vi "RT-Main.vi"   [LabVIEW 2019]
uses:
  <vilib>/nisyscfg/Close (System).vi
  <vilib>/nisyscfg/nisyscfg.lvlib
  <vilib>/NI_Real-Time Target Support.lvlib
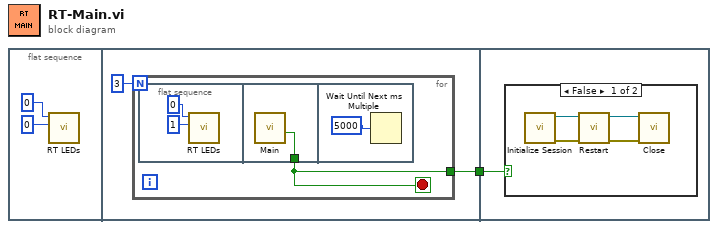
[diagram p0: block diagram]
diagram:
  n1 = flat-sequence {
    tunnel: [w4] -> w1
    tunnel: w1 -> [w11]
    frame #0 {
      n2 = call <vilib>:"RT LEDs.vi"("State"=0, "LED Num"=0 ("State")) -> ()  [unwired: 4 in, 2 out]
    }
    frame #1 {
      n3 = for {
        N: 3 -> [_]
        tunnel: [w6] -> w4
        stop <- w6 stop-if-true
        n4 = flat-sequence {
          tunnel: [w9] -> w6
          frame #0 {
            n5 = call <vilib>:"RT LEDs.vi"("State"=1, "LED Num"=0 ("State")) -> ()  [unwired: 4 in, 2 out]
          }
          frame #1 {
            n6 = call "Main.vi"() -> ("Aborted"=w9:bool)  [unwired: 10 in, 1 out]
          }
          frame #2 {
            n7 = Wait Until Next ms Multiple(millisecond multiple=u32 5000) -> ()  [unwired: 1 out]
          }
        }
      }
    }
    frame #2 {
      n8 = case shown="False" w11 {
        frame False {
          n9 = call <vilib>:"Initialize Session.vi"() -> ("error out"=w12:errorcluster, "Session out"=w15:refnum<k21>)  [unwired: 10 in]
          n10 = call <vilib>:"Restart.vi"("error in (no error)"=w12, "Session in"=w15) -> ("error out"=w14:errorcluster, "Session out"=w13:refnum<k21>)  [unwired: 7 in, 1 out]
          n11 = call-poly <vilib>:"Close.vi"("error in (no error)"=w14, "Session in"=w13) -> ()  [unwired: 9 in, 1 out]
        }
        frame True {
        }
      }
    }
  }
